vi "CONV 1D String Array to String.vi"(0 "1-D String":string[](array[string]), 1 "Delimiter (,)":string=",") -> (6 "String":string)   [LabVIEW 2017]
doc: "This routine converts a 1-D String Array into a String list. Delimiter may be one or more characters."
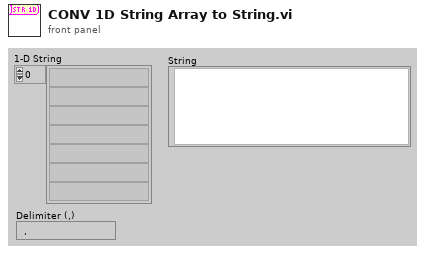
[diagram p1: front panel]
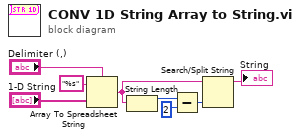
[diagram p0: block diagram]
diagram:
  n1 = Array To Spreadsheet String(delimiter (Tab)="Delimiter (,)", array="1-D String", 3:"%s" ("format string")) -> (spreadsheet string=w2:string)
  n2 = String Length(string=w2) -> (length=w4:i32)
  n3 = Subtract(x=w4, y=2) -> (x-y=w8:i32)
  n4 = Search/Split String(string=w2, offset (0)=w8) -> (substring before match=→"String":string)  [unwired: 3 out]
